vi "RandomMove.vi"(8 "error in (no error)":errorcluster caption="错误输入（无错误）", 9 "limit":dbl=40.0 format="%#_13g", 11 "RandomMoveBool 输入":refnum<class "RandomMoveBool.lvclass">) -> (0 "error out":errorcluster caption="错误输出", 3 "RandomMoveBool 输出":refnum<class "RandomMoveBool.lvclass">)   [LabVIEW 2018, in "RandomMoveBool.lvclass"]
uses:
  RandomMoveBool.lvclass
  <vilib>/Utility/miscctls.llb/LVPositionTypeDef.ctl
  RandomMoveBool.lvclass/RandomMoveBool.ctl
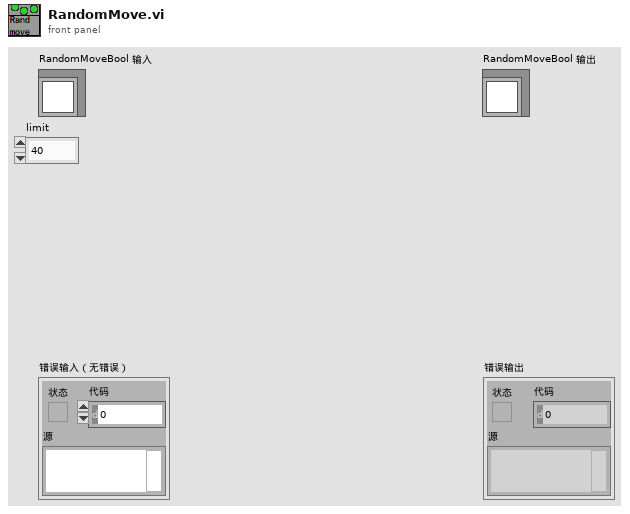
[diagram p1: front panel]
types:
  T1 = typedef "LVPositionTypeDef.ctl" = cluster{"Left":i32, "Top":i32}
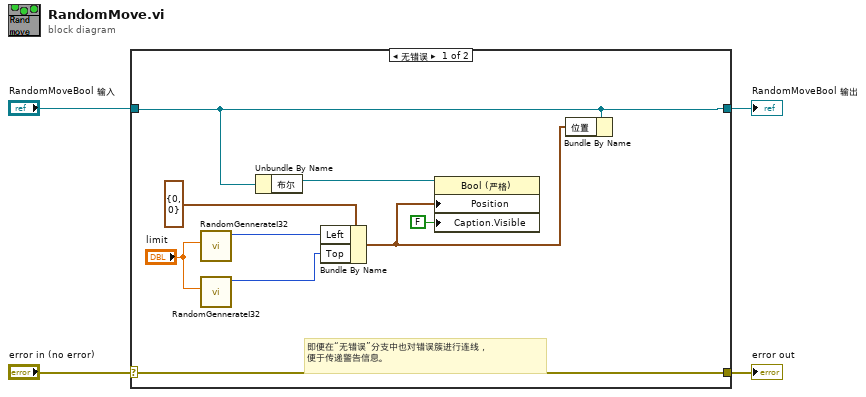
[diagram p0: block diagram]
diagram:
  n1 = case shown="无错误" "error in (no error)" {
    selector: "error in (no error)" -> [w13 w15]
    tunnel: [w13 w15] -> w3
    tunnel: [w11 w14] -> w1
    tunnel: "RandomMoveBool 输入" -> [w11 w14]
    frame No Error {
      # "即便在“无错误”分支中也对错误簇进行连线，\n便于传递警告信息。"
      n2 = call "RandomGennerateI32.vi"("limit"="limit") -> ("32位整型"=w9:i32)  [unwired: 10 in]
      n3 = call "RandomGennerateI32.vi"("limit"="limit") -> ("32位整型"=w8:i32)  [unwired: 10 in]
      n4 = Unbundle By Name(w11) -> ("布尔"=w12:refnum<vi>)
      n5 = Bundle By Name(cluster=T1 {"Left"=0, "Top"=0} ("位置"), "Left"=w9, "Top"=w8) -> (w7:T1)
      n6 = property class="Bool (严格)"(reference=w12, "Position"=w7, "Caption.Visible"=FALSE ("标题.可见")) -> ()  [unwired: 1 in, 2 out]
      n7 = Bundle By Name(cluster=w11, "位置"=w7) -> ()  [unwired: 1 out]
    }
    frame Error {
    }
  }
  "error out" <- w3
  "RandomMoveBool 输出" <- w1
